vi "robot_focus.vi"(1 "Buttons":T2, 2 "Parameters":T3={"Robot_vel"=0.3, "Robot_acc"=0.1, "Z-tolerance (mm)"=0.2, "Angle tolerance (deg)"=1.0, "frame_width"=500, "radius (mm)"=6.5, "angle_end (deg)"=0.0, "number of points"=18, "robot_ready"=FALSE, "z_height"=0.0, "X (mm)"=0.0, "Y (mm)"=0.0, "apply offset"=FALSE, "angle_start (deg)"=0.0, "N_OCT"=0, "apply_octa"=FALSE}, 3 "img":u8[][](array[numeric])) -> (0 "Output":T1)   [LabVIEW 2024]
panel:
  # "Robot Focus code"
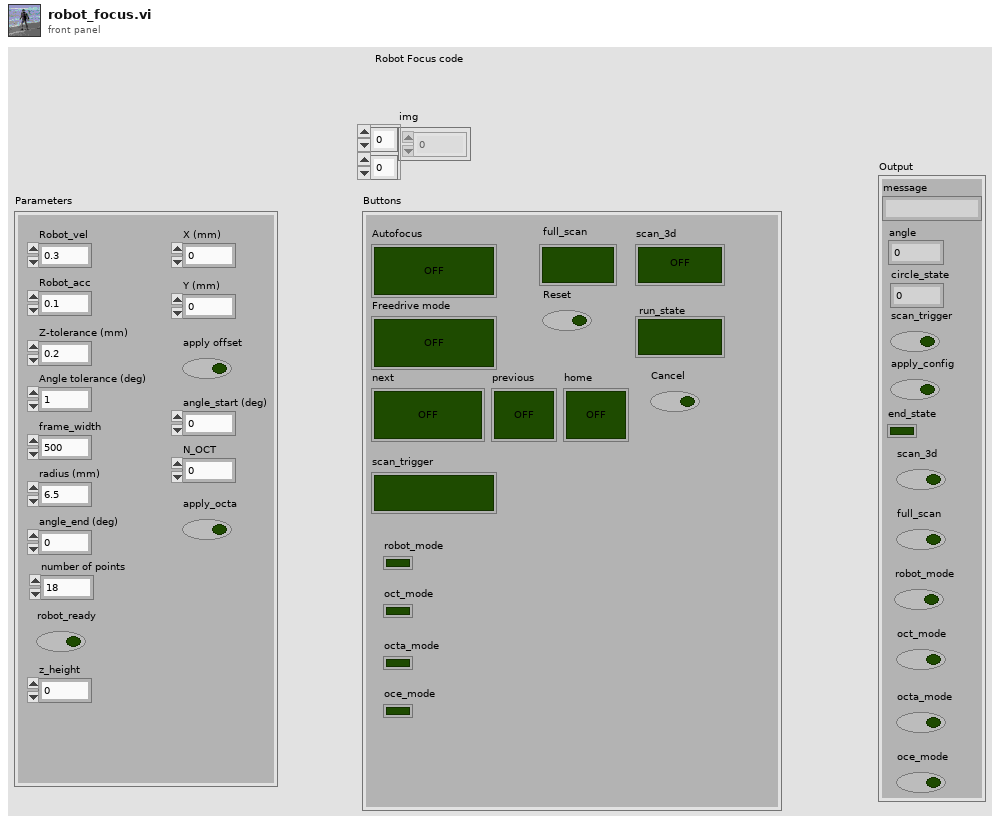
[diagram p1: front panel]
types:
  T1 = cluster{"message":string, "angle":dbl, "circle_state":dbl, "scan_trigger":bool, "apply_config":bool, "end_state":bool, "scan_3d":bool, "full_scan":bool, "robot_mode":bool, "oct_mode":bool, "octa_mode":bool, "oce_mode":bool}
  T2 = cluster{"Autofocus":bool, "Freedrive mode":bool, "next":bool, "previous":bool, "home":bool, "Reset":bool, "full_scan":bool, "scan_3d":bool, "run_state":bool, "Cancel":bool, "scan_trigger":bool, "robot_mode":bool, "oct_mode":bool, "octa_mode":bool, "oce_mode":bool}
  T3 = cluster{"Robot_vel":dbl, "Robot_acc":dbl, "Z-tolerance (mm)":dbl, "Angle tolerance (deg)":dbl, "frame_width":i16, "radius (mm)":dbl, "angle_end (deg)":dbl, "number of points":i32, "robot_ready":bool, "z_height":dbl, "X (mm)":dbl, "Y (mm)":dbl, "apply offset":bool, "angle_start (deg)":dbl, "N_OCT":i32, "apply_octa":bool}
  T4 = cluster{"img":u8[][], "Robot_vel":dbl, "Robot_acc":dbl, "Z-tolerance (mm)":dbl, "Angle tolerance (deg)":dbl, "frame_width":i16, "radius (mm)":dbl, "angle_end (deg)":dbl, "number of points":i32, "robot_ready":bool, "z_height":dbl, "X (mm)":dbl, "Y (mm)":dbl, "apply offset":bool, "angle_start (deg)":dbl, "N_OCT":i32, "apply_octa":bool}
  T5 = cluster{"msg":string, "angle":dbl, "circle_state":i32, "scan_trigger":bool, "apply_config":bool, "end_state":bool, "scan_3d":bool, "full_scan":bool, "robot_mode":bool, "oct_mode":bool, "octa_mode":bool, "oce_mode":bool}
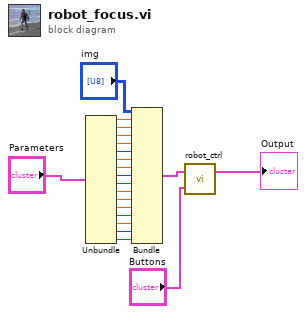
[diagram p0: block diagram]
diagram:
  n1 = Unbundle("Parameters") -> ("Robot_vel"=w17:dbl, "Robot_acc"=w16:dbl, "Z-tolerance (mm)"=w15:dbl, "Angle tolerance (deg)"=w14:dbl, "frame_width"=w13:i16, "radius (mm)"=w12:dbl, "angle_end (deg)"=w11:dbl, "number of points"=w10:i32, "robot_ready"=w9:bool, "z_height"=w8:dbl, "X (mm)"=w7:dbl, "Y (mm)"=w5:dbl, "apply offset"=w4:bool, "angle_start (deg)"=w3:dbl, "N_OCT"=w2:i32, "apply_octa"=w1:bool)
  n2 = Bundle("img"="img", "Robot_vel"=w17, "Robot_acc"=w16, "Z-tolerance (mm)"=w15, "Angle tolerance (deg)"=w14, "frame_width"=w13, "radius (mm)"=w12, "angle_end (deg)"=w11, "number of points"=w10, "robot_ready"=w9, "z_height"=w8, "X (mm)"=w7, "Y (mm)"=w5, "apply offset"=w4, "angle_start (deg)"=w3, "N_OCT"=w2, "apply_octa"=w1) -> (w19:T4)  [unwired: 1 in]
  n3 = call "robot_ctrl.vi"("Buttons"="Buttons", "Input"=w19) -> ("Output"=→"Output":T5)  [unwired: 1 in]
